vi "Rollover handler-Live protocols.vi"(9 "Tick Count Register in":u32=4000000000, 11 "Trigger delays":T1={"Trigger period in live protocols (80MHz Cycles)"=334000000, "Pulse width in live protocols (80MHz Cycles)"=0, "Enable stimulus in live protocols"=FALSE, "Trigger delay in funct. protocols (80MHz Cycles)"=400000, "Pulse width in funct. protocols (80MHz Cycles)"=400000, "Enable stimulus in funct. protocols"=FALSE}) -> (0 "Raw count":u32 caption="RAW Counter VI", 1 "Tick Count Register out":u32, 2 "Elapsed ticks count":u32, 3 "Target reached":bool)   [LabVIEW 2020]
uses:
  FPGA Typedefs/Stimulus trigger delays cluster.ctl
panel:
  # "304967295"
  # "Limited to 53.5 sec (if U32)"
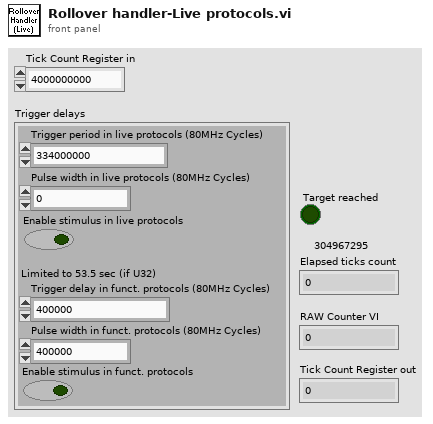
[diagram p1: front panel]
types:
  T1 = typedef "Stimulus trigger delays cluster.ctl" = cluster{"Trigger period in live protocols (80MHz Cycles)":u32, "Pulse width in live protocols (80MHz Cycles)":u32, "Enable stimulus in live protocols":bool, "Trigger delay in funct. protocols (80MHz Cycles)":u32, "Pulse width in funct. protocols (80MHz Cycles)":u32, "Enable stimulus in funct. protocols":bool}
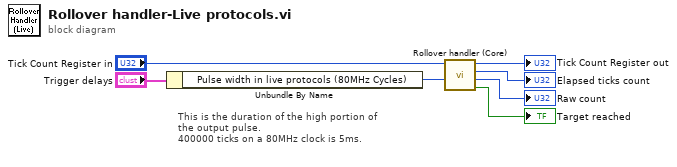
[diagram p0: block diagram]
diagram:
  # "This is the duration of the high portion of the output pulse.\n400000 ticks on a 80MHz clock is 5ms."
  n1 = Unbundle By Name("Trigger delays") -> ("Pulse width in live protocols (80MHz Cycles)"=w4:u32)
  n2 = call "Rollover handler (Core).vi"("Target delay"=w4, "Tick Count Register in"="Tick Count Register in") -> ("Target delay reached"=→"Target reached":bool, "Raw count"=→"Raw count":u32, "Elapsed ticks count"=→"Elapsed ticks count":u32, "Tick Count Register out"=→"Tick Count Register out":u32)  [unwired: 6 in]
